vi "Read.vi"(8 "error in (no error)":errorcluster, 11 "Class 1 in":refnum<class "csv.lvclass">) -> (0 "error out":errorcluster, 2 "Value":string, 3 "Class 1 out":refnum<class "csv.lvclass">)   [LabVIEW 2021, in "Library.lvlib" / "csv.lvclass"]
uses:
  csv.lvclass
  csv.lvclass/csv.ctl
  <vilib>/Utility/file.llb/Read Delimited Spreadsheet (string).vi
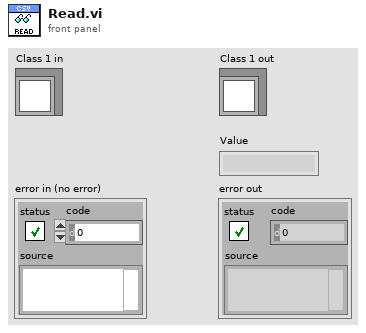
[diagram p1: front panel]
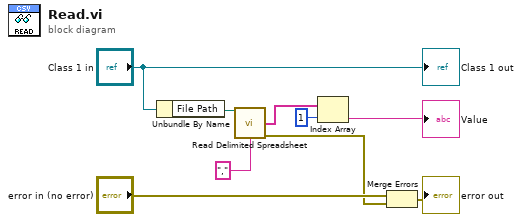
[diagram p0: block diagram]
diagram:
  n1 = Unbundle By Name("Class 1 in") -> ("File Path"=w7:path)
  n2 = call-poly <vilib>:"Read Delimited Spreadsheet.vi"("file path (dialog if empty)"=w7, "delimiter (\\t)"="," ("delimiter (\\t)")) -> ("first row"=w6:string[], "error out"=w3:errorcluster)  [unwired: 8 in, 4 out]
  n3 = Index Array(array=w6, index=1) -> (element=→"Value":string)
  n4 = Merge Errors("error in (no error)", w3) -> (→"error out":errorcluster)
  "Class 1 out" <- "Class 1 in"
